vi "CALC_FUNC_DOM_USER_STAR.vi"(0 "VISA IN":refnum<visa-resource-name>, 1 "Range number":i32, 2 "Start Value":i32, 5 "error in":errorcluster, 7 "Channel":i32) -> (14 "VISA Out":refnum<visa-resource-name>, 19 "error out":errorcluster)   [LabVIEW 2018, in "PNA-X.lvlib"]
doc: "CALCulate<cnum>:FUNCtion:DOMain:USER:STARt <range>, <start> \n(Read-Write) Sets the start of the specified user-domain range. \nTo apply this range, use CALC:FUNC:DOM:USER \nTo set the stop of the range, use CALC:FUNC:DOM:USER:STOP. \nSee Critical Note \nNote: This command does the same as CALC:MARK:FUNC:DOM:USER:STAR \nParameters \n<cnum> Channel number of the measurement. There must be a selected measurement \non that channel. If unspecified, <cnum> is set to 1. \n<range> Range number that will receive the start value. Choose an integer between 1 \nand 16 \n<start> Start value of the specified range. Choose a real number between: \nthe analyzer's Minimum and Maximum x-axis value. \nExamples CALC:FUNC:DOM:USER:STAR 1,1e9 \ncalculate2:function:domain:user:start 2,2e9 \n1517\n\nQuery Syntax CALCulate<cnum>:FUNCtion:DOMain:USER:STARt? <range> \nReturn Type Numeric \nDefault The analyzer's Minimum x-axis value"
uses:
  PNA-X.lvlib
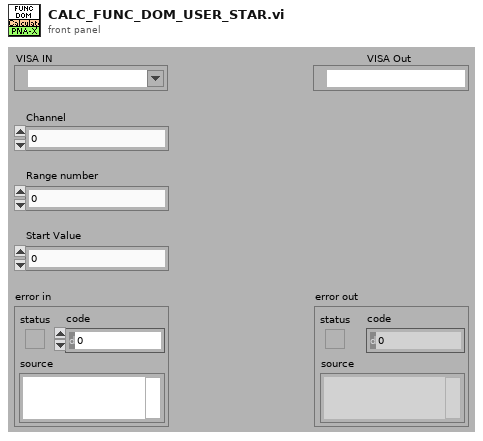
[diagram p1: front panel]
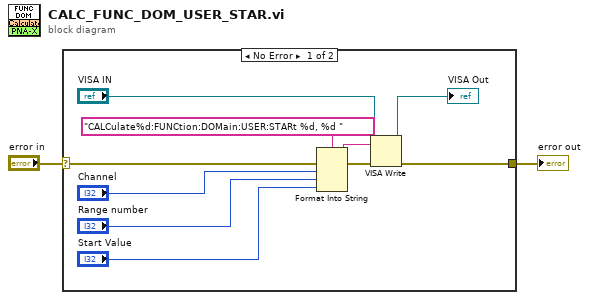
[diagram p0: block diagram]
diagram:
  n1 = case shown="No Error" "error in" {
    selector: "error in" -> [w12 w13]
    tunnel: [w7 w13] -> w1
    frame No Error {
      n2 = Format Into String(format string="CALCulate%d:FUNCtion:DOMain:USER:STARt %d, %d " ("Cmdline"), error in=w12, "Channel", "Range number", "Start Value") -> (resulting string=w10:string, error out=w11:errorcluster)  [unwired: 1 in]
      n3 = VISA Write(VISA resource name="VISA IN", write buffer=w10, error in (no error)=w11) -> (VISA resource name out=→"VISA Out":refnum<visa-resource-name>, error out=w7:errorcluster)  [unwired: 1 out]
    }
    frame Error {
    }
  }
  "error out" <- w1
